vi "initialise_controls.vi"(8 "error in (no error)":errorcluster, 11 "DataCollectionDL090215 in":refnum<class "DataCollectionDL090215.lvclass">) -> (0 "error out":errorcluster, 3 "DataCollectionDL090215 out":refnum<class "DataCollectionDL090215.lvclass">)   [LabVIEW 2010, in "DataCollectionDL090215.lvclass"]
uses:
  DataCollectionDL090215.lvclass
  DataCollectionDL090215.lvclass/DataCollectionDL090215.ctl
  common/classes/ErrorController/ErrorController/class_data.vi
  common/classes/ErrorController/ErrorController/ErrorController.lvclass
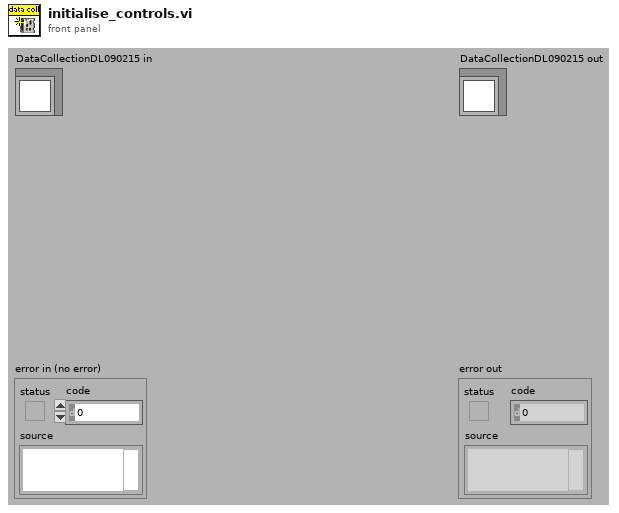
[diagram p1: front panel]
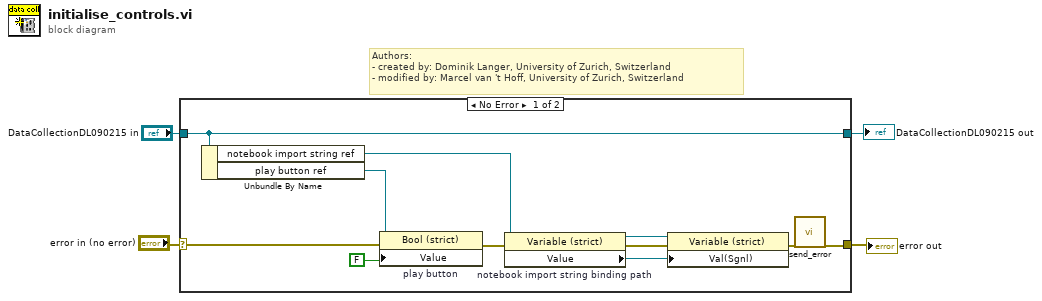
[diagram p0: block diagram]
diagram:
  # "Authors: \n- created by: Dominik Langer, University of Zurich, Switzerland\n- modified by: Marcel van 't Hoff, University of Zurich, Switzerland"
  n1 = case shown="No Error" "error in (no error)" {
    selector: "error in (no error)" -> [w9 w17]
    tunnel: [w14 w17] -> w1
    tunnel: [w7 w16] -> w2
    tunnel: "DataCollectionDL090215 in" -> [w7 w16]
    frame No Error {
      n2 = Unbundle By Name(w7) -> ("notebook import string ref"=w6:refnum<vi>, "play button ref"=w5:refnum<vi>)
      n3 = property on="play button" class="Bool (strict)"(reference=w5, error in=w9, "Value"=FALSE) -> (error out=w8:errorcluster)  [unwired: 1 out]
      n4 = property on="notebook import string binding path" class="Variable (strict)"(reference=w6, error in=w8) -> (reference out=w12:refnum<vi>, error out=w13:errorcluster, "Value"=w11:refnum<k21>)
      n5 = property class="Variable (strict)"(reference=w12, error in=w13, "Val(Sgnl)"=w11) -> (error out=w10:errorcluster)  [unwired: 1 out]
      n6 = call "send_error.vi"("error in (no error)"=w10) -> ("error out"=w14:errorcluster)  [unwired: 10 in]
    }
    frame Error {
    }
  }
  "error out" <- w1
  "DataCollectionDL090215 out" <- w2
